vi "Flatten Cluster To CfgTable(with DataName).vi"(5 "Format":string, 6 "Array delimiters (|)":string="|", 8 "error in (no error)":errorcluster, 10 "ParentName":string, 11 "Cluster Configuration Typedef":variant) -> (0 "error out":errorcluster, 2 "CfgTable Row Header":string[](array[string]), 3 "CfgTable Row":string[](array[string]))   [LabVIEW 2017, in "ClusterCfgTable.lvlib"]
doc: "Converts a cluster into a two-dimensional configuration table, naming each row after its data path below ParentName. Format and Array delimiters (|) control how values and array elements are written."
uses:
  ClusterCfgTable.lvlib
  <vilib>/Utility/Data Type/Type Definitions/Data Type.ctl
  <vilib>/Utility/Data Type/NI_Data Type.lvlib
  _openG/_reuse_openG.lvlib
panel:
  in  "ConfigStrings Typedef":string[](array[string])
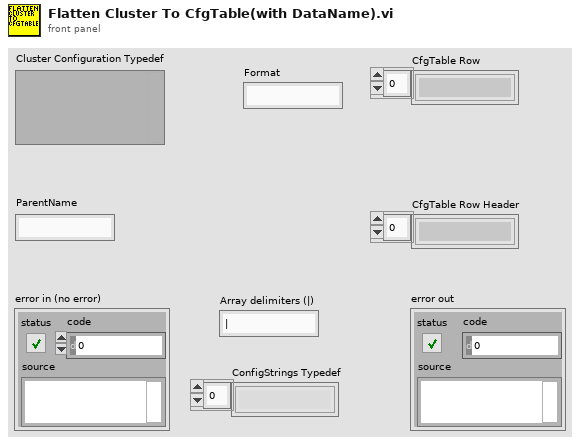
[diagram p1: front panel]
types:
  T1 = typedef "NI_Data Type.lvlib/Data Type.ctl" = enum8{"Invalid Type", "Void", "I8", "I16", "I32", "I64", "U8", "U16", "U32", "U64", "Single Float", "Double Float", "Extended Float", "Single Complex", "Double Complex", "Extended Complex", "Enum U8", "Enum U16", "Enum U32", "Enum U64", "Single Float With Unit", "Double Float With Unit", "Extended Float With Unit", "Single Complex with Unit", "Double Complex with Unit", "Extended Complex with Unit", "Boolean", "String", "Path", "Picture", "Tag", "Array", "Cluster", "Variant", "LV Variant", "Waveform", "Timestamp", "Digital Waveform", "Digital Data", "ExpressData", "Refnum", "External Data", "VI", "Poly VI", "LabVIEW Class Instance", "Fixed Point"}
  T2 = typedef "NI_Data Type.lvlib/Refnum Type.ctl" = enum16{"NotARefnum", "UnknownRefnum", "Generic", "Datalog", "ByteStream", "Device", "Occurence", "TCPNetConnection", "Auto", "Menu", "Imaq", "Hardware", "DataSocket", "Visa", "IVI", "UDPNetConnection", "Notifier", "Queue", "Irda", "EventReg", "DotNet", "UserEvent", "Callback", "UNUSED_EMPTY_POSITION", "BlueToothNetConnection", "LVObjApp", "LVObjVI", "LVObjUnknown", "GenericClass", "UserDefinedRefnumTag", "DataValue", "RT FIFO", "TDMS File"}
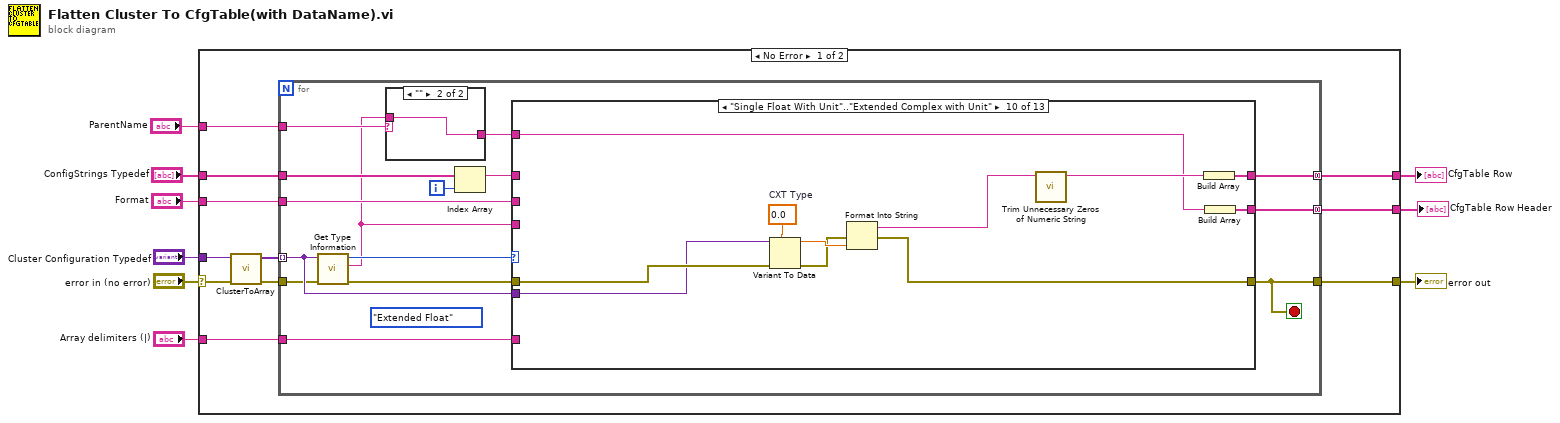
[diagram p0: block diagram]
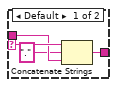
[diagram p2: hidden frame]
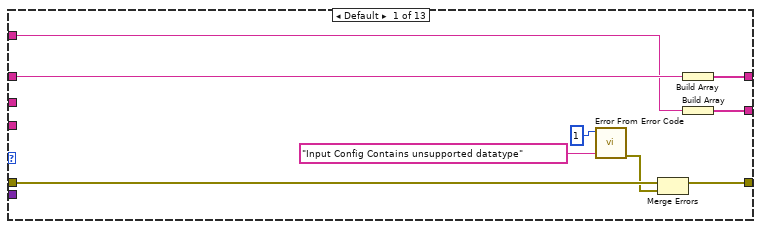
[diagram p3: hidden frame]
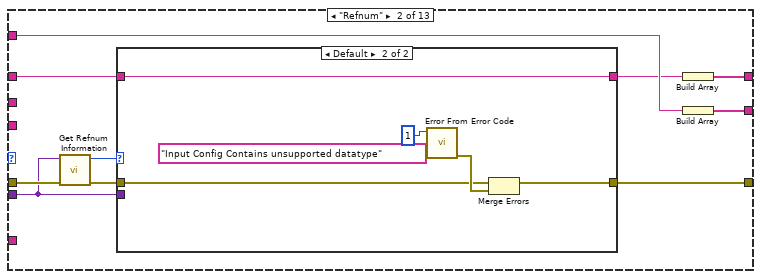
[diagram p4: hidden frame]
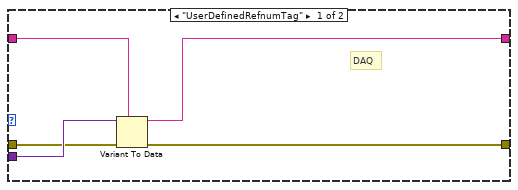
[diagram p5: hidden frame]
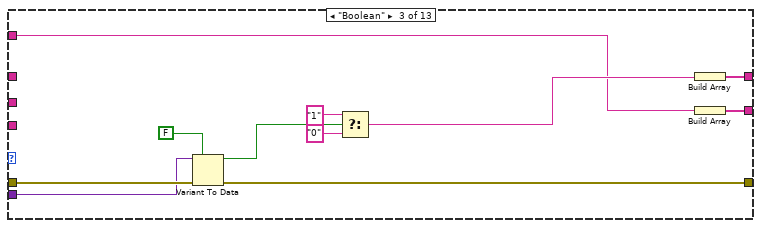
[diagram p6: hidden frame]
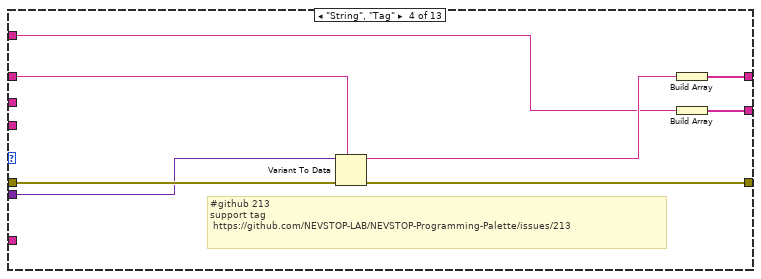
[diagram p7: hidden frame]
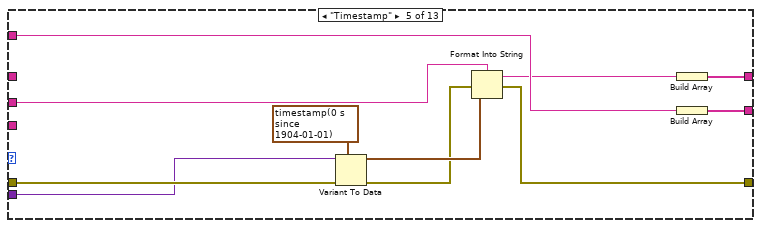
[diagram p8: hidden frame]
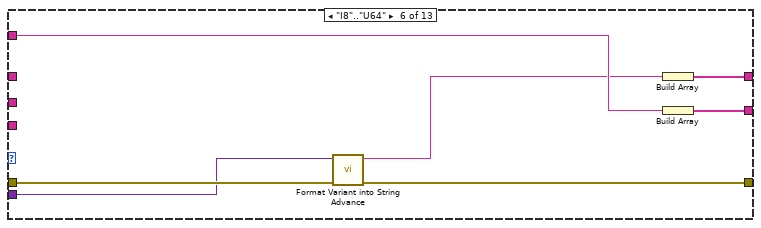
[diagram p9: hidden frame]
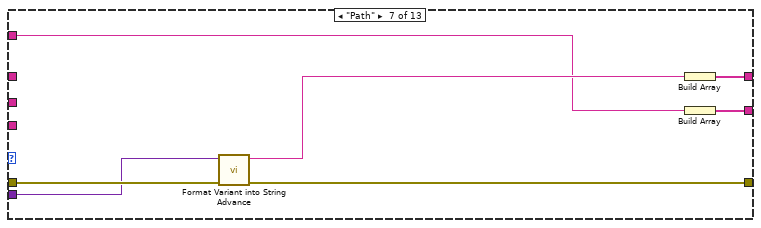
[diagram p10: hidden frame]
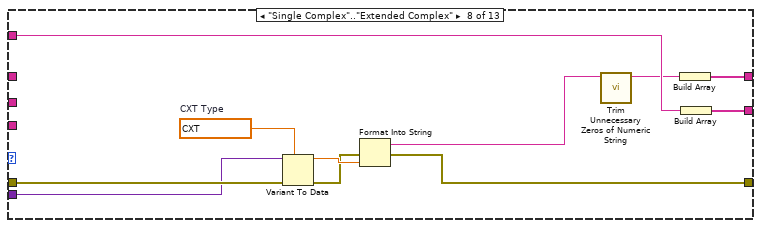
[diagram p11: hidden frame]
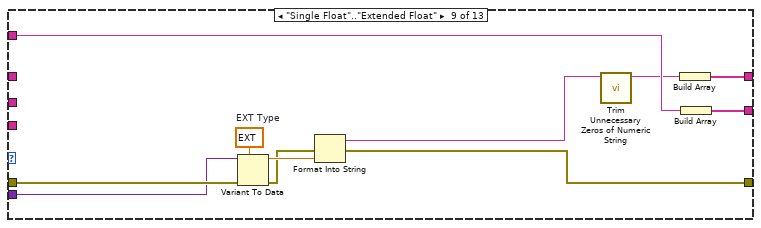
[diagram p12: hidden frame]
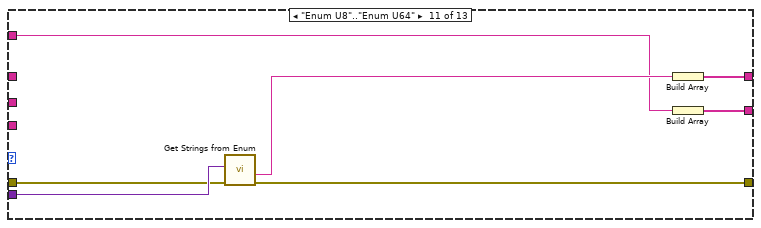
[diagram p13: hidden frame]
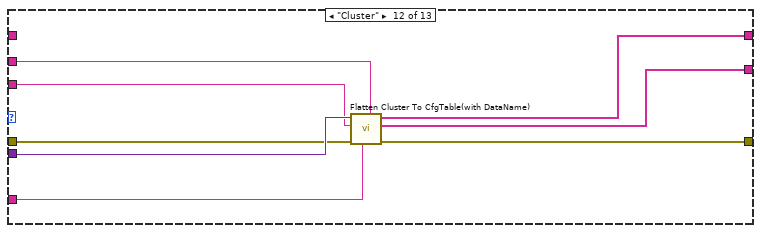
[diagram p14: hidden frame]
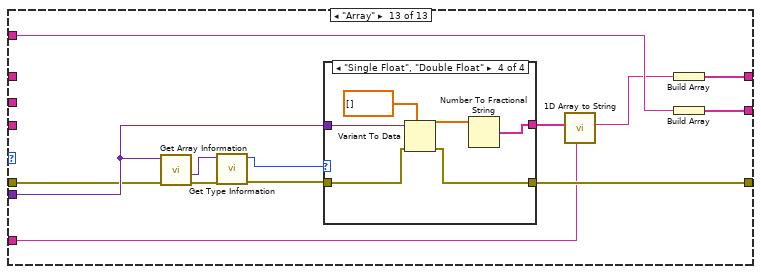
[diagram p15: hidden frame]
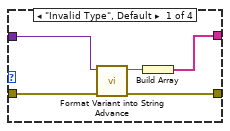
[diagram p16: hidden frame]
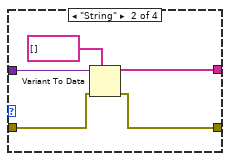
[diagram p17: hidden frame]
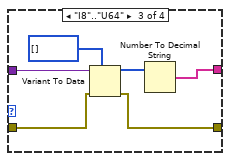
[diagram p18: hidden frame]
diagram:
  n1 = case shown="No Error" "error in (no error)" {
    selector: "error in (no error)" -> [w18 w199]
    tunnel: [w20 w199] -> w9
    tunnel: "Cluster Configuration Typedef" -> [w16 _]
    tunnel: [w15 w198] -> w6
    tunnel: "ConfigStrings Typedef" -> [w14 w198]
    tunnel: "ParentName" -> [w13 _]
    tunnel: [w12 _] -> w3
    tunnel: "Array delimiters (|)" -> [w11 _]
    tunnel: "Format" -> [w10 _]
    frame No Error {
      n2 = call "ClusterToArray.vi"("Error in"=w18, "Cluster"=w16) -> ("Error out"=w19:errorcluster, "Array"=w17:variant[])  [unwired: 8 in]
      n3 = for {
        tunnel: w17 -> [w23] mode=indexing
        tunnel: w19 -> [w22]
        tunnel: [w34] -> w20
        tunnel: [w33] -> w15 mode=concatenating
        tunnel: w14 -> [w32]
        tunnel: w13 -> [w29]
        tunnel: [w27] -> w12 mode=concatenating
        tunnel: w11 -> [w26]
        tunnel: w10 -> [w24]
        i -> [w30]
        stop <- w34 stop-if-true
        (unwired) Data_Type."Extended Float" ("Type")
        n4 = call <vilib>:"Get Type Information.vi"("error in (no error)"=w22, "Variant"=w23) -> ("error out"=w25:errorcluster, "Name"=w21:string, "Type"=w35:T1)  [unwired: 5 in, 2 out]
        n5 = case shown="\"\"" w29 {
          selector: w29 -> [w39 _]
          tunnel: w21 -> [w38 w40]
          tunnel: [w36 w40] -> w28
          frame Default {
            n6 = Concatenate Strings(w39, "." ("string"), w38) -> (w36:string)
          }
          frame "" {
          }
        }
        n7 = Index Array(array=w32, index=w30) -> (element=w31:string)
        n8 = case shown="\"Single Float With Unit\"..\"Extended Complex with Unit\"" w35 {
          tunnel: w23 -> [_ w52 w80 w87 w99 w102 w108 w116 w128 w139 w154 w162 w170]
          tunnel: w25 -> [w49 w59 w81 w89 w100 w103 w114 w117 w129 w140 w153 w160 w167]
          tunnel: [w48 w58 w78 w88 w90 w104 w113 w118 w126 w138 w151 w159 w172] -> w34
          tunnel: [w43 w57 w77 w84 w98 w107 w111 w125 w136 w146 w150 w161 w175] -> w33
          tunnel: w31 -> [w44 w51 _ w86 _ _ _ _ _ _ _ _ _]
          tunnel: w21 -> [_ _ _ _ _ _ _ _ _ _ _ w158 _]
          tunnel: w28 -> [w42 w56 w76 w83 w97 w106 w110 w124 w135 w145 w149 _ w174]
          tunnel: [w41 w55 w75 w82 w96 w105 w109 w123 w134 w144 w148 w157 w173] -> w27
          tunnel: w26 -> [_ _ _ _ _ _ _ _ _ _ _ w156 w168]
          tunnel: w24 -> [_ _ _ _ w92 _ _ _ _ _ _ w155 _]
          frame Default {
            n9 = call "Error From Error Code.vi"("error message (\"\")"="Input Config Contains unsupported datatype" ("String to Prepend to source (\"\")"), "error code (0)"=1 ("code")) -> ("error out"=w47:errorcluster)  [unwired: 7 in]
            n10 = Merge Errors(w49, w47) -> (w48:errorcluster)
            n11 = Build Array(w44) -> (w43:string[])
            n12 = Build Array(w42) -> (w41:string[])
          }
          frame "Refnum" {
            n13 = call <vilib>:"Get Refnum Information.vi"("error in (no error)"=w59, "Variant"=w52) -> ("error out"=w54:errorcluster, "Reference Type"=w53:T2)  [unwired: 6 in, 2 out]
            n14 = case shown="Default" w53 {
              tunnel: [w60 w70] -> w58
              tunnel: w54 -> [w63 w66]
              tunnel: w52 -> [w64 _]
              tunnel: w51 -> [w62 w65]
              tunnel: [w61 w65] -> w50
              frame "UserDefinedRefnumTag" {
                # "DAQ"
                n15 = Variant To Data(error in=w63, type=w62, Variant=w64) -> (data=w61:string, error out=w60:errorcluster)
              }
              frame Default {
                n16 = call "Error From Error Code.vi"("error message (\"\")"="Input Config Contains unsupported datatype" ("String to Prepend to source (\"\")"), "error code (0)"=1 ("code")) -> ("error out"=w69:errorcluster)  [unwired: 7 in]
                n17 = Merge Errors(w66, w69) -> (w70:errorcluster)
              }
            }
            n18 = Build Array(w50) -> (w57:string[])
            n19 = Build Array(w56) -> (w55:string[])
          }
          frame "Boolean" {
            n20 = Variant To Data(error in=w81, type=FALSE, Variant=w80) -> (data=w73:bool, error out=w78:errorcluster)
            n21 = Select(t="1", s=w73, f="0") -> (s? t:f=w79:string)
            n22 = Build Array(w79) -> (w77:string[])
            n23 = Build Array(w76) -> (w75:string[])
          }
          frame "String", "Tag" {
            # "#github 213\nsupport tag\n https://github.com/NEVSTOP-LAB/NEVSTOP-Programming-Palette/issues/213"
            n24 = Variant To Data(error in=w89, type=w86, Variant=w87) -> (data=w85:string, error out=w88:errorcluster)
            n25 = Build Array(w85) -> (w84:string[])
            n26 = Build Array(w83) -> (w82:string[])
          }
          frame "Timestamp" {
            n27 = Variant To Data(error in=w100, type=timestamp(0 s since 1904-01-01), Variant=w99) -> (data=w94:timestamp, error out=w91:errorcluster)
            n28 = Format Into String(format string=w92, error in=w91, w94) -> (resulting string=w93:string, error out=w90:errorcluster)  [unwired: 1 in]
            n29 = Build Array(w93) -> (w98:string[])
            n30 = Build Array(w97) -> (w96:string[])
          }
          frame "I8".."U64" {
            n31 = call "Format Variant into String Advance.vi"("error in (no error)"=w103, "Variant"=w102) -> ("error out"=w104:errorcluster, "Data"=w101:string)  [unwired: 7 in, 1 out]
            n32 = Build Array(w101) -> (w107:string[])
            n33 = Build Array(w106) -> (w105:string[])
          }
          frame "Path" {
            n34 = call "Format Variant into String Advance.vi"("error in (no error)"=w114, "Variant"=w108) -> ("error out"=w113:errorcluster, "Data"=w112:string)  [unwired: 7 in, 1 out]
            n35 = Build Array(w112) -> (w111:string[])
            n36 = Build Array(w110) -> (w109:string[])
          }
          frame "Single Complex".."Extended Complex" {
            w121 = cxt 0.0+0.0i  # CXT Type
            n37 = Variant To Data(error in=w117, type=w121, Variant=w116) -> (data=w120:cxt, error out=w119:errorcluster)
            n38 = Format Into String(error in=w119, w120) -> (resulting string=w115:string, error out=w118:errorcluster)  [unwired: 2 in]
            n39 = call "Trim Unnecessary Zeros of Numeric String.vi"("Output String in"=w115) -> ("Output String out"=w122:string)  [unwired: 10 in]
            n40 = Build Array(w122) -> (w125:string[])
            n41 = Build Array(w124) -> (w123:string[])
          }
          frame "Single Float".."Extended Float" {
            w132 = ext 0.0  # EXT Type
            n42 = Variant To Data(error in=w129, type=w132, Variant=w128) -> (data=w131:ext, error out=w130:errorcluster)
            n43 = Format Into String(error in=w130, w131) -> (resulting string=w127:string, error out=w126:errorcluster)  [unwired: 2 in]
            n44 = call "Trim Unnecessary Zeros of Numeric String.vi"("Output String in"=w127) -> ("Output String out"=w133:string)  [unwired: 10 in]
            n45 = Build Array(w133) -> (w136:string[])
            n46 = Build Array(w135) -> (w134:string[])
          }
          frame "Single Float With Unit".."Extended Complex with Unit" {
            w143 = 0.0  # CXT Type
            n47 = Variant To Data(error in=w140, type=w143, Variant=w139) -> (data=w142:dbl, error out=w141:errorcluster)
            n48 = Format Into String(error in=w141, w142) -> (resulting string=w137:string, error out=w138:errorcluster)  [unwired: 2 in]
            n49 = call "Trim Unnecessary Zeros of Numeric String.vi"("Output String in"=w137) -> ("Output String out"=w147:string)  [unwired: 10 in]
            n50 = Build Array(w147) -> (w146:string[])
            n51 = Build Array(w145) -> (w144:string[])
          }
          frame "Enum U8".."Enum U64" {
            n52 = call "Get Strings from Enum.vi"("error in (no error)"=w153, "Enum"=w154) -> ("error out"=w151:errorcluster, "String Value"=w152:string)  [unwired: 6 in, 2 out]
            n53 = Build Array(w152) -> (w150:string[])
            n54 = Build Array(w149) -> (w148:string[])
          }
          frame "Cluster" {
            n55 = call "Flatten Cluster To CfgTable(with DataName).vi"("Format"=w155, "Array delimiters (|)"=w156, "error in (no error)"=w160, "ParentName"=w158, "Cluster Configuration Typedef"=w162) -> ("error out"=w159:errorcluster, "CfgTable Row Header"=w157:string[], "CfgTable Row"=w161:string[])  [unwired: 4 in]
          }
          frame "Array" {
            n56 = call <vilib>:"Get Array Information.vi"("error in (no error)"=w167, "Variant"=w170) -> ("error out"=w166:errorcluster, "Array Element Data Type"=w164:variant)  [unwired: 6 in, 2 out]
            n57 = call <vilib>:"Get Type Information.vi"("error in (no error)"=w166, "Variant"=w164) -> ("error out"=w165:errorcluster, "Type"=w163:T1)  [unwired: 5 in, 3 out]
            n58 = case shown="\"Single Float\", \"Double Float\"" w163 {
              tunnel: [w176 w181 w186 w192] -> w171
              tunnel: [w179 w183 w189 w195] -> w172
              tunnel: w165 -> [w180 w184 w190 w196]
              tunnel: w170 -> [w178 w185 w191 w197]
              frame "Invalid Type", Default {
                n59 = call "Format Variant into String Advance.vi"("error in (no error)"=w180, "Variant"=w178) -> ("error out"=w179:errorcluster, "Data"=w177:string)  [unwired: 7 in, 1 out]
                n60 = Build Array(w177) -> (w176:string[])
              }
              frame "String" {
                n61 = Variant To Data(error in=w184, type=string[] [] ("Data"), Variant=w185) -> (data=w181:string[], error out=w183:errorcluster)
              }
              frame "I8".."U64" {
                n62 = Variant To Data(error in=w190, type=i32[] [] ("Data"), Variant=w191) -> (data=w187:i32[], error out=w189:errorcluster)
                n63 = Number To Decimal String(number=w187) -> (decimal integer string=w186:string[])  [unwired: 1 in]
              }
              frame "Single Float", "Double Float" {
                n64 = Variant To Data(error in=w196, type=dbl[] [] ("Data"), Variant=w197) -> (data=w193:dbl[], error out=w195:errorcluster)
                n65 = Number To Fractional String(number=w193) -> (F-format string=w192:string[])  [unwired: 3 in]
              }
            }
            n66 = call "1D Array to String.vi"("delimiter (Tab)"=w168, "Array of Strings"=w171) -> ("delimited string"=w169:string)  [unwired: 9 in]
            n67 = Build Array(w169) -> (w175:string[])
            n68 = Build Array(w174) -> (w173:string[])
          }
        }
      }
    }
    frame Error {
    }
  }
  "CfgTable Row" <- w6
  "error out" <- w9
  "CfgTable Row Header" <- w3
